vi "Close Run.vi"(8 "error in (no error)":errorcluster, 11 "xwpfRun in":refnum<class "xwpfRun.lvclass">) -> (0 "error out":errorcluster, 3 "xwpfRun out":refnum<class "xwpfRun.lvclass">)   [LabVIEW 2017, in "Word_Specific.lvlib" / "xwpfRun.lvclass"]
uses:
  xwpfRun.lvclass
  xwpfRun.lvclass/xwpfRun.ctl
  Get Run Ref.vi
  C:/Users/Neo/Desktop/Dev_Tools_BR/LabVIEW_NPOI/src/lib/NPOI 2.1.1/NPOI.OOXML.dll
  lib/NPOI 2.1.1/NPOI.OOXML.dll
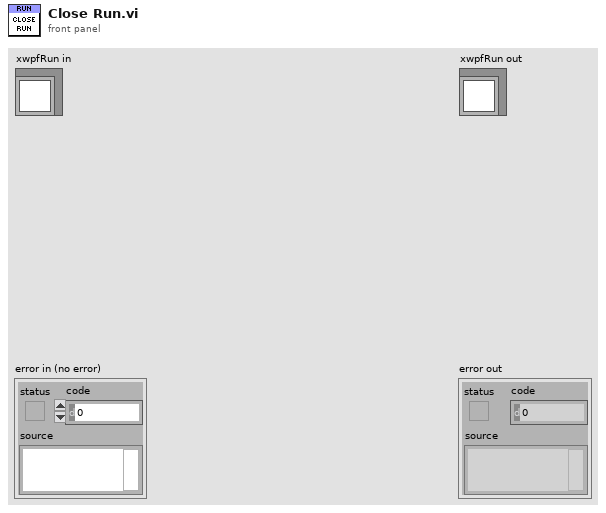
[diagram p1: front panel]
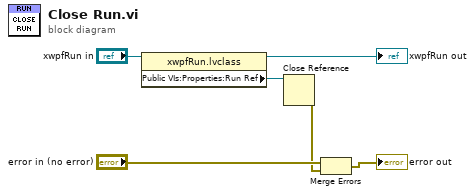
[diagram p0: block diagram]
diagram:
  n1 = property class="xwpfRun.lvclass"(reference="xwpfRun in") -> (reference out=→"xwpfRun out":refnum<class "xwpfRun.lvclass">, "Public VIs:Properties:Run Ref"=w3:refnum<k24>)  [unwired: 1 in, 1 out]
  n2 = Close Reference(reference=w3) -> (error out=w1:errorcluster)  [unwired: 1 in]
  n3 = Merge Errors("error in (no error)", w1) -> (→"error out":errorcluster)
